vi "Handle Error.vi"(8 "error in (no error)":errorcluster, 11 "CS++RTMainActor in":refnum<class "CS++RTMainActor.lvclass">) -> (0 "error out":errorcluster, 2 "stop actor?":bool=TRUE, 3 "CS++RTMainActor out":refnum<class "CS++RTMainActor.lvclass">)   [LabVIEW 2014, in "CS++RTMain.lvlib" / "CS++RTMainActor.lvclass"]
doc: "(<B>Filename</B>: Actor Framework.lvlib:Actor.lvclass:Handle Error.vi)\n\nDefines how the actor handles an error that occurred while processing a message. By default, this method does nothing except stop the actor."
uses:
  CS++RTMainActor.lvclass
  CSPP_Core/Libraries/Base/Severity.ctl
  CS++RTMainActor.lvclass/CS++RTMainActor.ctl
  CS++RTMainActor Messages/LNA Return Message Msg/LNA Return Message Msg.lvclass
  <vilib>/ActorFramework/Actor/Actor.lvclass/Actor.ctl
  <vilib>/ActorFramework/Message Enqueuer/Message Enqueuer.lvclass/Message Enqueuer.ctl
  <vilib>/ActorFramework/Message Enqueuer/Init from Existing Queue.vi
  <vilib>/ActorFramework/Message Enqueuer/Message Enqueuer.lvclass
  <vilib>/ActorFramework/Actor/Actor.lvclass
  CSPP_LNA/CS++LNA.lvlib
  CSPP_Core/Libraries/Utilities/CS++Utilities.lvlib
  CSPP_Core/Libraries/Base/CS++Base.lvlib
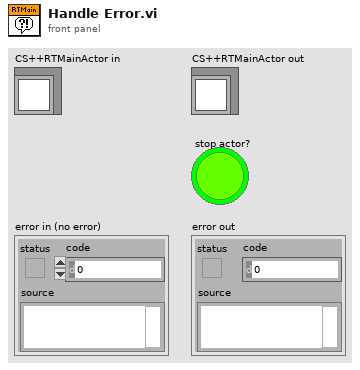
[diagram p1: front panel]
types:
  T1 = typedef "CS++Base.lvlib/Severity.ctl" = enum16{"emergency", "alert", "critical", "error", "warning", "notice", "info", "debug"}
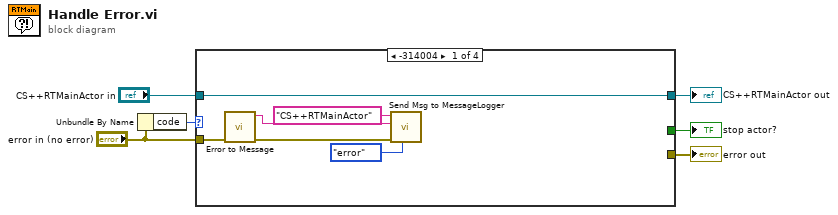
[diagram p0: block diagram]
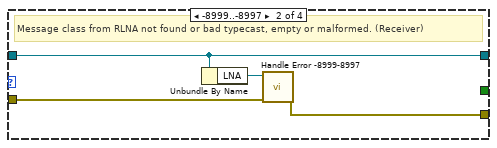
[diagram p2: hidden frame]
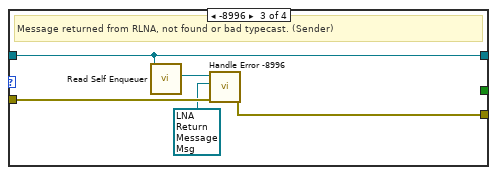
[diagram p3: hidden frame]
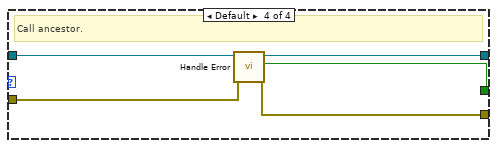
[diagram p4: hidden frame]
diagram:
  n1 = Unbundle By Name("error in (no error)") -> ("code"=w6:i32)
  n2 = case shown="-314004" w6 {
    tunnel: [_ w13 w19 w24] -> w3
    tunnel: [w12 w16 w21 w23] -> w1
    tunnel: "error in (no error)" -> [w11 w14 w18 w25]
    tunnel: "CS++RTMainActor in" -> [w12 w16 w21 w26]
    tunnel: [_ _ _ w22] -> w2
    frame -314004 {
      n3 = call "Error to Message.vi"("Error In"=w11) -> ("Error Out"=w8:errorcluster, "Error Message"=w10:string)  [unwired: 9 in]
      n4 = call "Send Msg to MessageLogger.vi"("Severity Code (info)"=Severity."error", "Error In"=w8, "Message Content"=w10, "Message Tag"="CS++RTMainActor") -> ()  [unwired: 7 in, 1 out]
    }
    frame -8999..-8997 {
      # "Message class from RLNA not found or bad typecast, empty or malformed. (Receiver)"
      n5 = Unbundle By Name(w16) -> ("LNA"=w15:refnum<class "Message Enqueuer.lvclass">)
      n6 = call "Handle Error -8999-8997.vi"("Tx Error"=w14, "Message Enqueuer in"=w15) -> ("Error Out"=w13:errorcluster)  [unwired: 9 in]
    }
    frame -8996 {
      # "Message returned from RLNA, not found or bad typecast. (Sender)"
      n7 = call <vilib>:"Read Self Enqueuer.vi"("Actor"=w21) -> ("Self Enqueuer"=w20:refnum<class "Message Enqueuer.lvclass">)  [unwired: 10 in]
      n8 = call "Handle Error -8996.vi"("Tx Error"=w18, "LNA Return Message Msg"=refnum<class "LNA Return Message Msg.lvclass"> refnum ("CS++RTMain.lvlib:LNA Return Message Msg.lvclass"), "Message Enqueuer in"=w20) -> ("Error Out"=w19:errorcluster)  [unwired: 8 in]
    }
    frame Default {
      # "Call ancestor."
      n9 = call-parent "Handle Error.vi"("error in (no error)"=w25, "Actor in"=w26) -> ("error out"=w24:errorcluster, "stop actor?"=w22:bool, "Actor out"=w23:refnum<class "CS++RTMainActor.lvclass">)  [unwired: 7 in]
    }
  }
  "CS++RTMainActor out" <- w1
  "error out" <- w3
  "stop actor?" <- w2
